vi "subvi_tick_distance_conversion.vi"(6 "distance/count":dbl, 9 "Acceleration (Counts/Interval)":i32, 10 "Velocity (Counts/Interval)":i32, 11 "Position (Counts)":i64) -> (1 "Acceleration [length/time^2]":dbl format="%.2f", 2 "Velocity [length/time]":dbl format="%.2f", 3 "Position [length]":dbl)   [LabVIEW 2019]
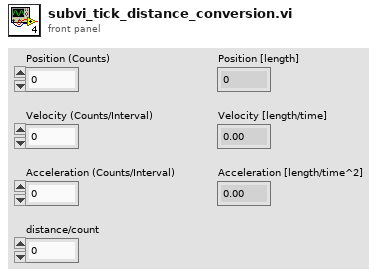
[diagram p1: front panel]
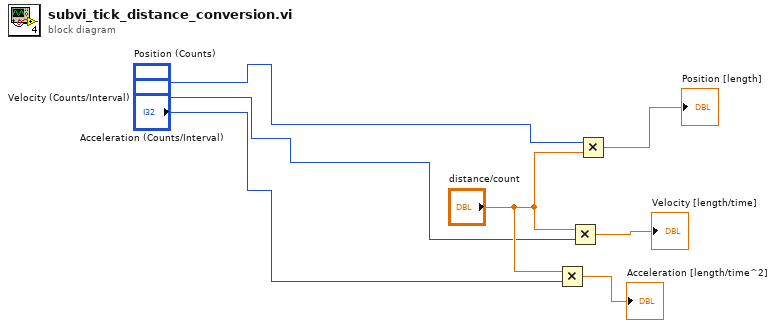
[diagram p0: block diagram]
diagram:
  n1 = Multiply(x="distance/count", y="Acceleration (Counts/Interval)") -> (x*y=→"Acceleration [length/time^2]":dbl)
  n2 = Multiply(x="distance/count", y="Velocity (Counts/Interval)") -> (x*y=→"Velocity [length/time]":dbl)
  n3 = Multiply(x="Position (Counts)", y="distance/count") -> (x*y=→"Position [length]":dbl)
